vi "smsAvlCode (SubVI).vi"(0 "Iniciar":T5, 1 "Password":string, 2 "APN":T3, 3 "IP/Port":T4, 4 "DNS":T2, 5 "GPRS":bool, 6 "Intervalo":T1, 7 "I/O":bool, 10 "Comando":u16(ring)=5 items=["Password", "APN", "IP/Port", "DNS", "GPRS", "Intervalo", "I/O"]) -> ()   [LabVIEW 2012]
panel:
  out "concatenated string":string
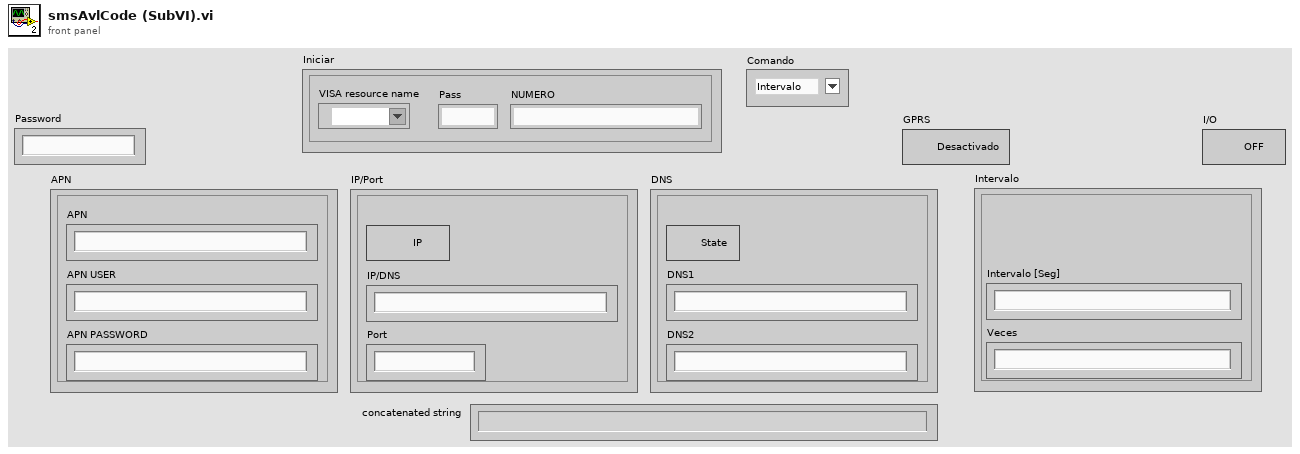
[diagram p1: front panel]
types:
  T1 = cluster{"Veces":string, "Intervalo [Seg]":string}
  T2 = cluster{"State":bool, "DNS2":string, "DNS1":string}
  T3 = cluster{"APN":string, "APN USER":string, "APN PASSWORD":string}
  T4 = cluster{"ip dns":bool, "IP/DNS":string, "Port":string}
  T5 = cluster{"VISA resource name":refnum<visa-resource-name>, "Pass":string, "NUMERO":string}
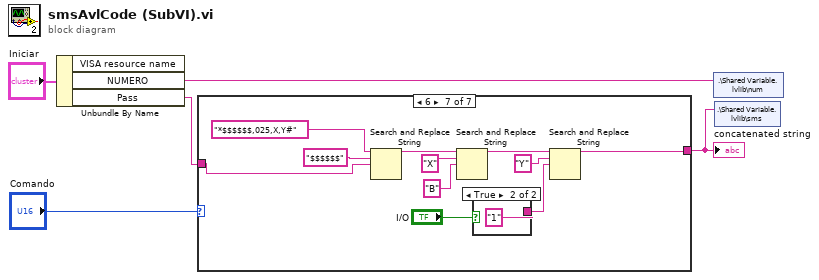
[diagram p0: block diagram]
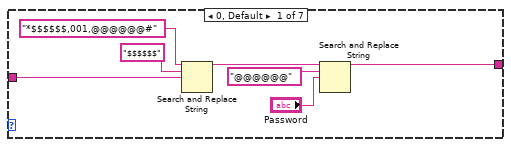
[diagram p2: hidden frame]
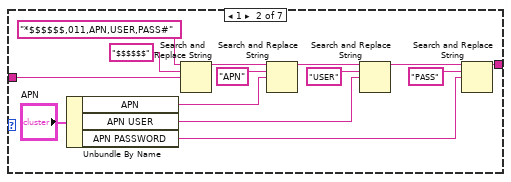
[diagram p3: hidden frame]
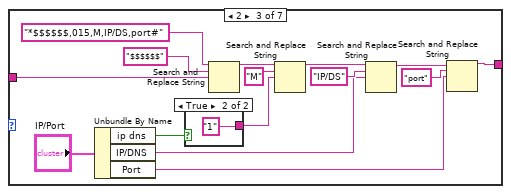
[diagram p4: hidden frame]
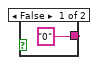
[diagram p5: hidden frame]
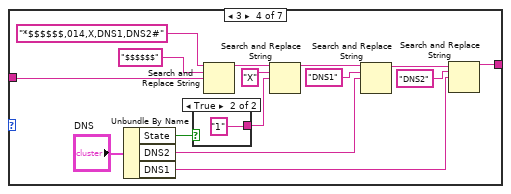
[diagram p6: hidden frame]
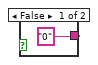
[diagram p7: hidden frame]
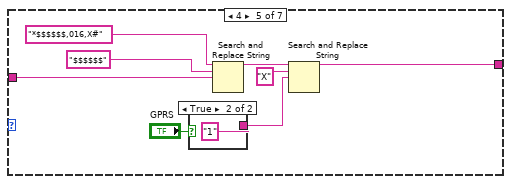
[diagram p8: hidden frame]
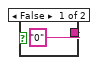
[diagram p9: hidden frame]
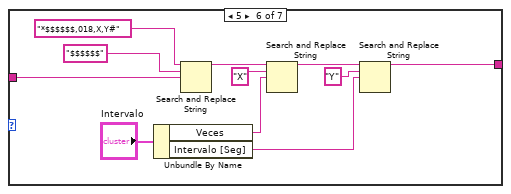
[diagram p10: hidden frame]
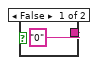
[diagram p11: hidden frame]
diagram:
  n1 = Unbundle By Name("Iniciar") -> ("NUMERO"=w1:string, "Pass"=w3:string)  [unwired: 1 out]
  n2 = case shown="6" "Comando" {
    tunnel: w3 -> [w8 w22 w31 w50 w66 w75 w85]
    tunnel: [w7 w17 w32 w49 w62 w74 w84] -> w2
    frame 0, Default {
      n3 = Search and Replace String(input string="*$$$$$$,001,@@@@@@#", search string="$$$$$$", replace string=w8) -> (result string=w6:string)  [unwired: 5 in, 3 out]
      n4 = Search and Replace String(input string=w6, search string="@@@@@@", replace string="Password") -> (result string=w7:string)  [unwired: 5 in, 3 out]
    }
    frame 1 {
      n5 = Unbundle By Name("APN") -> ("APN"=w15:string, "APN USER"=w14:string, "APN PASSWORD"=w13:string)
      n6 = Search and Replace String(input string="*$$$$$$,011,APN,USER,PASS#", search string="$$$$$$", replace string=w22) -> (result string=w23:string)  [unwired: 5 in, 3 out]
      n7 = Search and Replace String(input string=w23, search string="APN", replace string=w15) -> (result string=w20:string)  [unwired: 5 in, 3 out]
      n8 = Search and Replace String(input string=w20, search string="USER", replace string=w14) -> (result string=w18:string)  [unwired: 5 in, 3 out]
      n9 = Search and Replace String(input string=w18, search string="PASS", replace string=w13) -> (result string=w17:string)  [unwired: 5 in, 3 out]
    }
    frame 2 {
      n10 = Unbundle By Name("IP/Port") -> ("ip dns"=w29:bool, "IP/DNS"=w28:string, "Port"=w27:string)
      n11 = case shown="True" w29 {
        tunnel: ["0" ("search string") "1" ("search string")] -> w33
        frame False {
        }
        frame True {
        }
      }
      n12 = Search and Replace String(input string="*$$$$$$,015,M,IP/DS,port#", search string="$$$$$$", replace string=w31) -> (result string=w38:string)  [unwired: 5 in, 3 out]
      n13 = Search and Replace String(input string=w38, search string="M", replace string=w33) -> (result string=w36:string)  [unwired: 5 in, 3 out]
      n14 = Search and Replace String(input string=w36, search string="IP/DS", replace string=w28) -> (result string=w35:string)  [unwired: 5 in, 3 out]
      n15 = Search and Replace String(input string=w35, search string="port", replace string=w27) -> (result string=w32:string)  [unwired: 5 in, 3 out]
    }
    frame 3 {
      n16 = Unbundle By Name("DNS") -> ("State"=w44:bool, "DNS2"=w47:string, "DNS1"=w46:string)
      n17 = case shown="True" w44 {
        tunnel: ["0" ("search string") "1" ("search string")] -> w45
        frame False {
        }
        frame True {
        }
      }
      n18 = Search and Replace String(input string="*$$$$$$,014,X,DNS1,DNS2#", search string="$$$$$$", replace string=w50) -> (result string=w55:string)  [unwired: 5 in, 3 out]
      n19 = Search and Replace String(input string=w55, search string="X", replace string=w45) -> (result string=w53:string)  [unwired: 5 in, 3 out]
      n20 = Search and Replace String(input string=w53, search string="DNS1", replace string=w47) -> (result string=w52:string)  [unwired: 5 in, 3 out]
      n21 = Search and Replace String(input string=w52, search string="DNS2", replace string=w46) -> (result string=w49:string)  [unwired: 5 in, 3 out]
    }
    frame 4 {
      n22 = case shown="True" "GPRS" {
        tunnel: ["0" ("search string") "1" ("search string")] -> w63
        frame False {
        }
        frame True {
        }
      }
      n23 = Search and Replace String(input string="*$$$$$$,016,X#", search string="$$$$$$", replace string=w66) -> (result string=w65:string)  [unwired: 5 in, 3 out]
      n24 = Search and Replace String(input string=w65, search string="X", replace string=w63) -> (result string=w62:string)  [unwired: 5 in, 3 out]
    }
    frame 5 {
      n25 = Unbundle By Name("Intervalo") -> ("Veces"=w72:string, "Intervalo [Seg]"=w71:string)
      n26 = Search and Replace String(input string="*$$$$$$,018,X,Y#", search string="$$$$$$", replace string=w75) -> (result string=w79:string)  [unwired: 5 in, 3 out]
      n27 = Search and Replace String(input string=w79, search string="X", replace string=w72) -> (result string=w81:string)  [unwired: 5 in, 3 out]
      n28 = Search and Replace String(input string=w81, search string="Y", replace string=w71) -> (result string=w74:string)  [unwired: 5 in, 3 out]
    }
    frame 6 {
      n29 = Search and Replace String(input string="*$$$$$$,025,X,Y#", search string="$$$$$$", replace string=w85) -> (result string=w90:string)  [unwired: 5 in, 3 out]
      n30 = Search and Replace String(input string=w90, search string="X", replace string="B" ("Intervalo [Seg] 2")) -> (result string=w92:string)  [unwired: 5 in, 3 out]
      n31 = case shown="True" "I/O" {
        tunnel: ["0" ("search string") "1" ("search string")] -> w83
        frame False {
        }
        frame True {
        }
      }
      n32 = Search and Replace String(input string=w92, search string="Y", replace string=w83) -> (result string=w84:string)  [unwired: 5 in, 3 out]
    }
  }
  "concatenated string" <- w2
  n33 = shared-variable ".\\Shared Variable.lvlib\\num"(w1) -> ()  [unwired: 1 in, 1 out]
  n34 = shared-variable ".\\Shared Variable.lvlib\\sms"(w2) -> ()  [unwired: 1 in, 1 out]
